vi "XCtlBlinkingLEDFacade.vi"(0 "Data In":T4, 2 "Display State In":T2, 3 "Container State":T3) -> (6 "Data Out":T4, 7 "Display State Out":T2, 8 "Action":T1)   [LabVIEW 2012, in "XCtlBlinkingLED.xctl"]
uses:
  XCtlBlinkingLED.xctl
  XCtlBlinkingLEDData.ctl
  <vilib>/_xctls/Container State.ctl
  XCtlBlinkingLEDState.ctl
  <vilib>/_xctls/Action.ctl
  <vilib>/_xctls/XControlSupport.lvlib
panel:
  out "BlinkingLED":bool
  # "This file is part of the package BlinkingLED.\n\nLicensed under the BSD license.\n\nCopyright (C) 2009, Martin Weiss.\nAll rights reserverd."
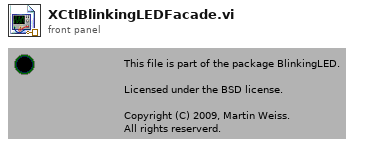
[diagram p1: front panel]
types:
  T1 = typedef "XControlSupport.lvlib/Action.ctl" = cluster{"Data Changed?":bool, "State Changed?":bool, "Action Name":string}
  T2 = typedef "XCtlBlinkingLED.xctl/XCtlBlinkingLEDState.ctl" = cluster{"Numeric":dbl}
  T3 = typedef "XControlSupport.lvlib/Container State.ctl" = cluster{"Indicator?":bool, "Run Mode?":bool, " Refnum":refnum<vi>}
  T4 = typedef "XCtlBlinkingLED.xctl/XCtlBlinkingLEDData.ctl" = i32
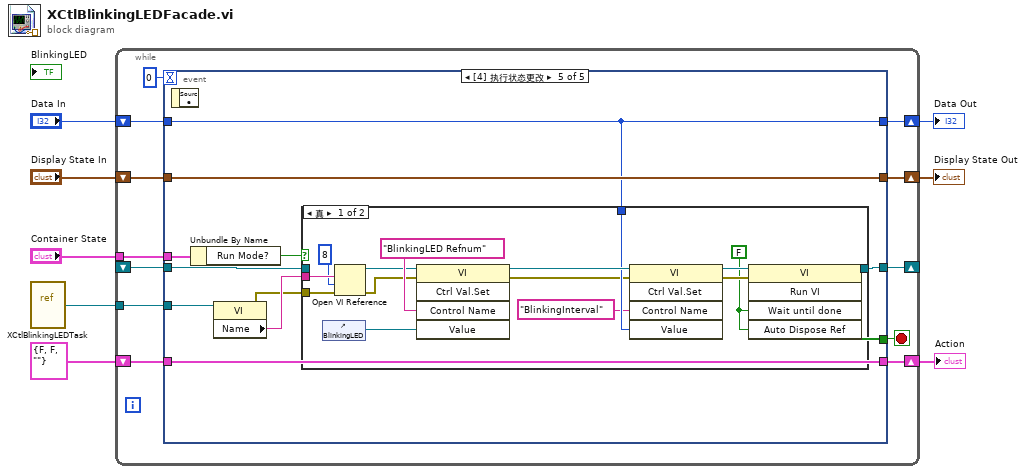
[diagram p0: block diagram]
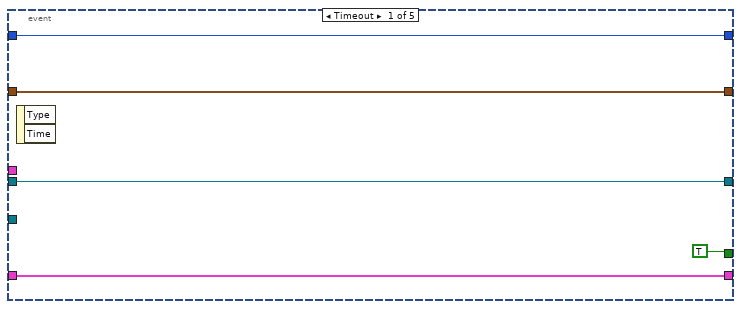
[diagram p2: hidden frame]
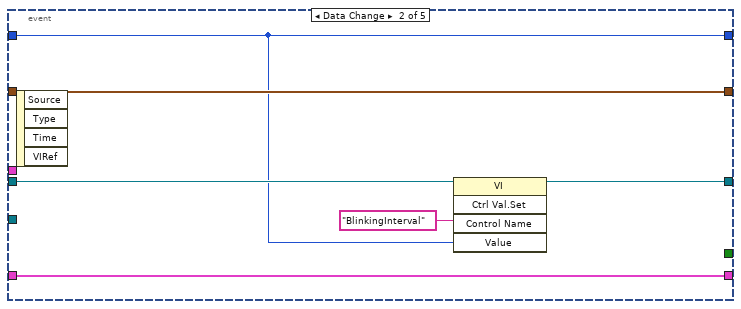
[diagram p3: hidden frame]
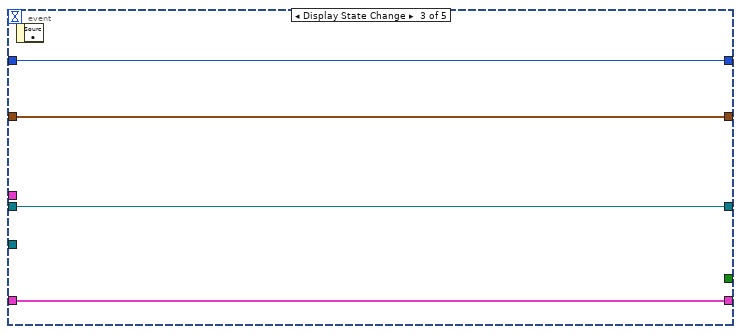
[diagram p4: hidden frame]
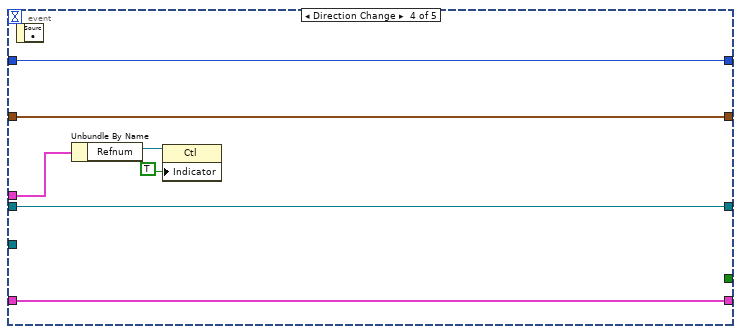
[diagram p5: hidden frame]
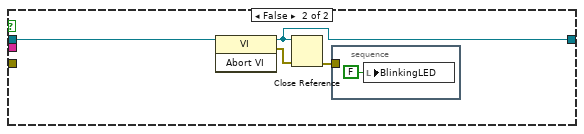
[diagram p6: hidden frame]
diagram:
  n1 = vi-ref "XCtlBlinkingLEDTask.vi"() -> (w1:refnum<vi>)
  n2 = while {
    shift-right: [w19] -> w5
    shift-left: "Display State In" -> [w20]
    tunnel: "Container State" -> [w16]
    shift-right: [w14] -> w8
    shift-left: "Data In" -> [w15]
    shift-right: [w12] -> w3
    shift-left: T1 {"Data Changed?"=FALSE, "State Changed?"=FALSE, "Action Name"=""} ("Action") -> [w13]
    shift-right: [w10] -> _
    shift-left: _ -> [w11]
    tunnel: w1 -> [w9]
    stop <- w18 stop-if-true
    n3 = event shown="[4] 执行状态更改" {
      selector: _ -> [_ _ _ _ _]
      dyn-events: _ -> [_ _ _ _ _]
      timeout: 0 -> [_ _ _ _ _]
      tunnel: w20 -> [w23 w31 w35 w41 w51]
      tunnel: [w23 w31 w35 w41 w51] -> w19
      tunnel: [TRUE _ _ _ _] -> w18
      tunnel: w16 -> [_ _ _ w42 w52]
      tunnel: w15 -> [w22 w27 w34 w40 w50]
      tunnel: [w22 w27 w34 w40 w50] -> w14
      tunnel: [w24 w30 w33 w39 w44] -> w12
      tunnel: w13 -> [w24 w30 w33 w39 w44]
      tunnel: w11 -> [w21 w28 w32 w38 w48]
      tunnel: [w21 w26 w32 w38 w49] -> w10
      tunnel: w9 -> [_ _ _ _ w47]
      event Timeout {
        n4 = event-data() -> ()  [unwired: 1 in, 2 out]
      }
      event Data Change {
        n5 = event-data() -> ()  [unwired: 1 in, 4 out]
        n6 = invoke class="VI" method="Ctrl Val.Set"(reference=w28, "Control Name"="BlinkingInterval", "Value"=w27) -> (reference out=w26:refnum<vi>)  [unwired: 2 in, 4 out]
      }
      event Display State Change {
        n7 = event-data() -> ()  [unwired: 1 in, 1 out]
      }
      event Direction Change {
        n8 = event-data() -> ()  [unwired: 1 in, 1 out]
        n9 = Unbundle By Name(w42) -> ("Refnum"=w37:refnum<vi>)
        n10 = property class="Ctl"(reference=w37, "Indicator"=TRUE) -> ()  [unwired: 1 in, 2 out]
      }
      event Exec State Change {
        n11 = event-data() -> ()  [unwired: 1 in, 1 out]
        n12 = Unbundle By Name(w52) -> ("Run Mode?"=w43:bool)
        n13 = property class="VI"(reference=w47) -> (error out=w45:errorcluster, "Name"=w46:string)  [unwired: 1 in, 1 out]
        n14 = case shown="真" w43 {
          tunnel: w50 -> [w65 _]
          tunnel: [w58 w69] -> w49
          tunnel: w48 -> [_ w71]
          tunnel: w46 -> [w56 _]
          tunnel: w45 -> [w54 _]
          frame True {
            w53 = FALSE ("结束前等待")
            n15 = control-ref of="BlinkingLED"() -> (w59:refnum<vi>)
            n16 = Open VI Reference(vi path=w56, options=8, error in (no error)=w54) -> (vi reference=w60:refnum<vi>, error out=w57:errorcluster)  [unwired: 3 in]
            n17 = invoke class="VI" method="Ctrl Val.Set"(reference=w60, error in=w57, "Control Name"="BlinkingLED Refnum", "Value"=w59) -> (reference out=w66:refnum<vi>, error out=w62:errorcluster)  [unwired: 1 in, 3 out]
            n18 = invoke class="VI" method="Ctrl Val.Set"(reference=w66, error in=w62, "Control Name"="BlinkingInterval", "Value"=w65) -> (reference out=w67:refnum<vi>, error out=w61:errorcluster)  [unwired: 1 in, 3 out]
            n19 = invoke class="VI" method="Run VI"(reference=w67, error in=w61, "Wait until done"=w53, "Auto Dispose Ref"=w53) -> (reference out=w58:refnum<vi>)  [unwired: 1 in, 4 out]
          }
          frame False {
            n20 = invoke class="VI" method="Abort VI"(reference=w71) -> (reference out=w69:refnum<vi>, error out=w70:errorcluster)  [unwired: 2 in, 1 out]
            n21 = Close Reference(reference=w69, error in (no error)=w70) -> (error out=w68:errorcluster)
            n22 = stacked-sequence {
              tunnel: w68 -> [_]
              frame #0 {
                n23 = local write "BlinkingLED"(FALSE ("BlinkingLED")) -> ()
              }
            }
          }
        }
      }
    }
  }
  "Display State Out" <- w5
  "Data Out" <- w8
  "Action" <- w3
